vi "vms_cancelCallback_command_standby.vi"(8 "error in (no error)":errorcluster) -> (0 "error out":errorcluster, 3 "function return":i32)   [LabVIEW 2016, in "SALLV_vms.lvlib"]
doc: "int vms_shm_cancelCallback_command_standbyLV();"
uses:
  SALLV_vms.lvlib
  SALLV_vms.so
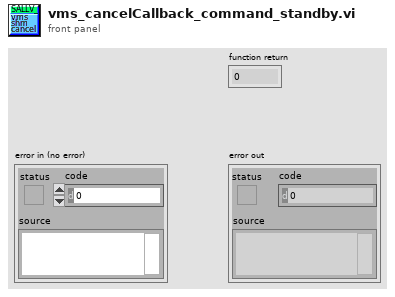
[diagram p1: front panel]
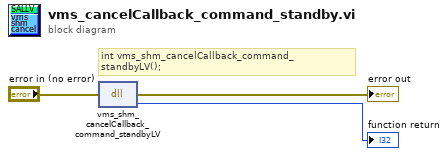
[diagram p0: block diagram]
diagram:
  # "int vms_shm_cancelCallback_command_standbyLV();"
  n1 = dll-call lib="opt/CODE/SALLV_vms/SALLV_vms.*" fn="vms_shm_cancelCallback_command_standbyLV"(error in="error in (no error)") -> (error out=→"error out":errorcluster, →"function return":i32)  [unwired: 2 in, 1 out]
